vi "the end - 복사본.vi"() -> ()   [LabVIEW 2011]
uses:
  <vilib>/NXT/Block Support/NXT_InputPort.ctl
  <vilib>/NXT/Subs/MotorOutput.ctl
  <vilib>/NXT/Dual Mode Library/Waits/Wait_Num.vi
  <vilib>/NXT/Dual Mode Library/Motors/MotorOn.vi
panel:
  out "Yes / No":bool
  in  "터치 센서 (port 2)":T1 caption="Port (Port 1)" items=["Port 1", "Port 2", "Port 3", "Port 4"]
  in  "소나 센서 (port 3)":T1=3 caption="Port (Port 4)" items=["Port 1", "Port 2", "Port 3", "Port 4"]
  in  "회전 각도 4":i32=180
  in  "회전 각도 3":i32=180
  in  "회전 포트 4":T2=3 items=["Port A"=0, "Port B"=1, "Port C"=2, "Ports A & B"=4, "Ports A & C"=5, "Ports B & C"=6, "All Ports"=3]
  in  "회전 포트 3":T2=3 items=["Port A"=0, "Port B"=1, "Port C"=2, "Ports A & B"=4, "Ports A & C"=5, "Ports B & C"=6, "All Ports"=3]
  in  "후진 시간 2":sgl=1.0
  in  "빛 센서 (port 1)":T1=2 caption="Port (Port 3)" items=["Port 1", "Port 2", "Port 3", "Port 4"]
  in  "정지":bool
  in  "회전 각도 2":i32=180
  in  "회전 각도 1":i32=180
  in  "회전 포트 1":T2=3 items=["Port A"=0, "Port B"=1, "Port C"=2, "Ports A & B"=4, "Ports A & C"=5, "Ports B & C"=6, "All Ports"=3]
  in  "회전 포트 2":T2=3 items=["Port A"=0, "Port B"=1, "Port C"=2, "Ports A & B"=4, "Ports A & C"=5, "Ports B & C"=6, "All Ports"=3]
  in  "후진 시간":sgl=1.0
  in  "Power (100)":i32=75
  in  "Output Port (All Ports)":T2=3 items=["Port A"=0, "Port B"=1, "Port C"=2, "Ports A & B"=4, "Ports A & C"=5, "Ports B & C"=6, "All Ports"=3]
  in  "빛 센서 (port 4)":T1=2 caption="Port (Port 3)" items=["Port 1", "Port 2", "Port 3", "Port 4"]
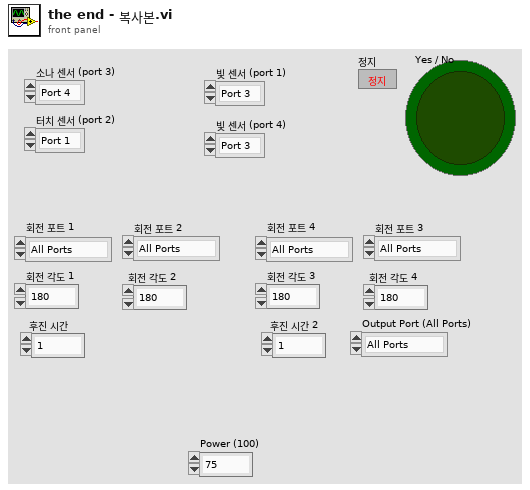
[diagram p1: front panel]
types:
  T1 = typedef "NXT_InputPort.ctl" = u8
  T2 = typedef "MotorOutput.ctl" = u8
  T3 = typedef "LVHSConnector.ctl" = cluster{"Hardware":string, "Flattened String":string}
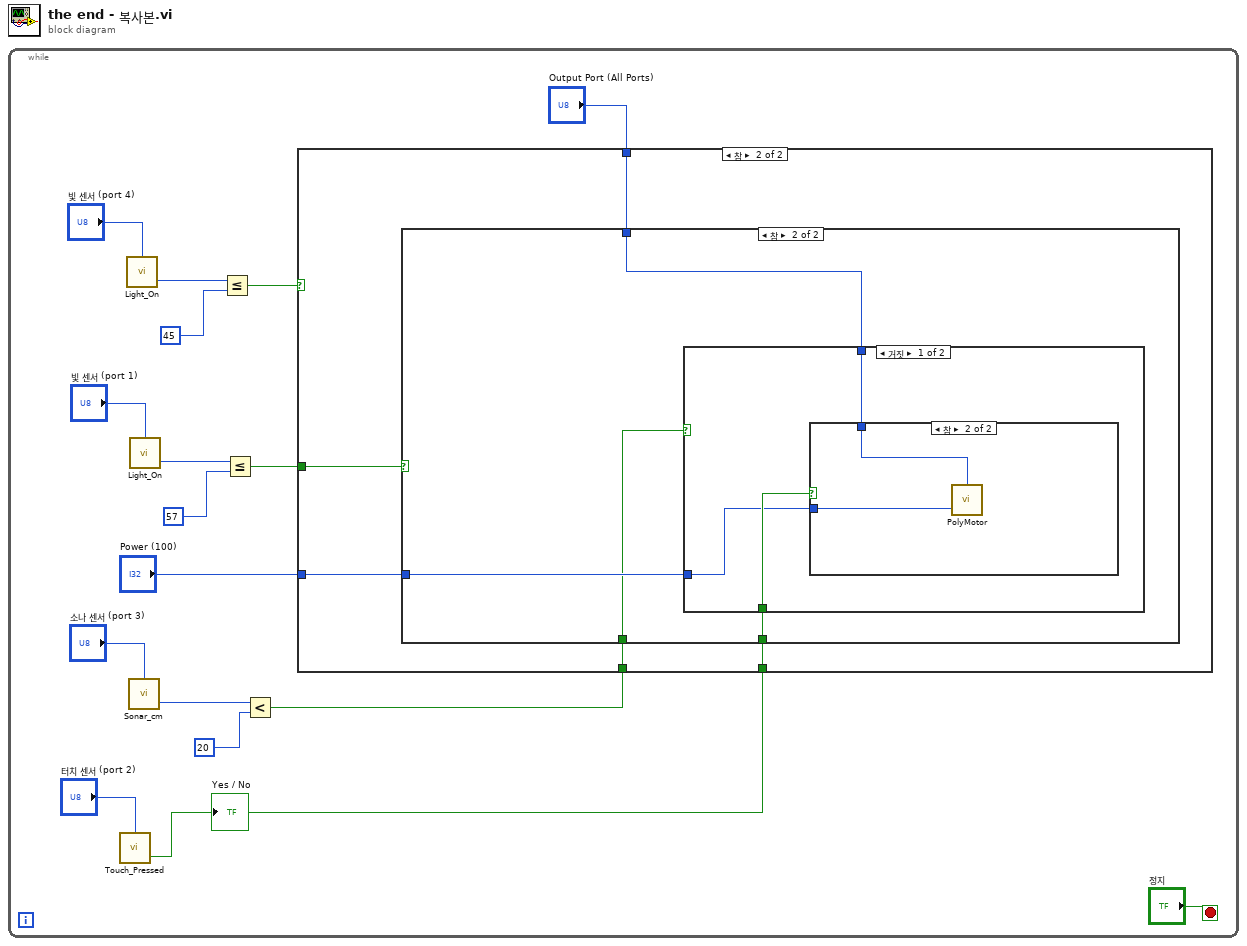
[diagram p0: block diagram]
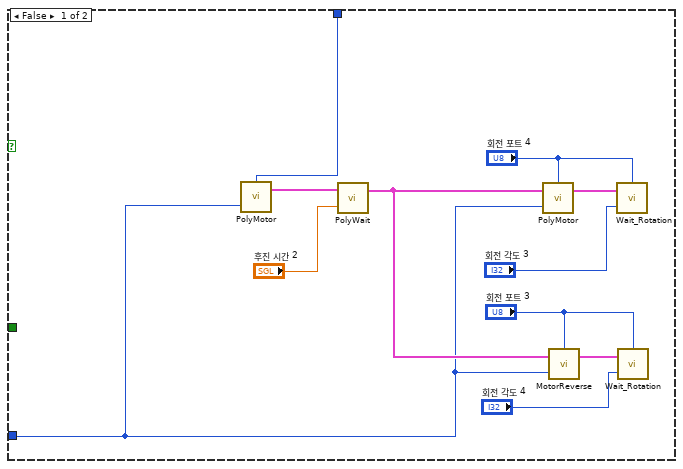
[diagram p2: hidden frame]
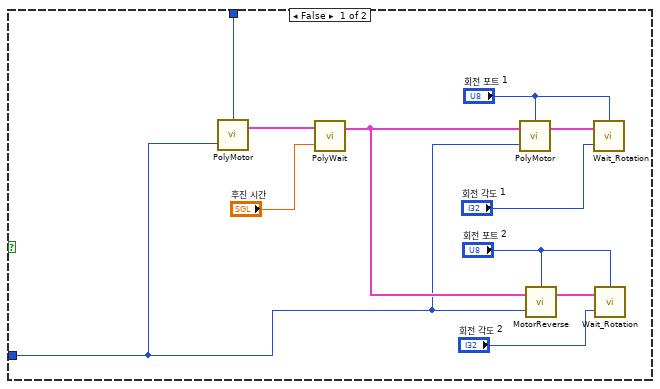
[diagram p3: hidden frame]
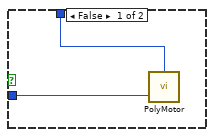
[diagram p4: hidden frame]
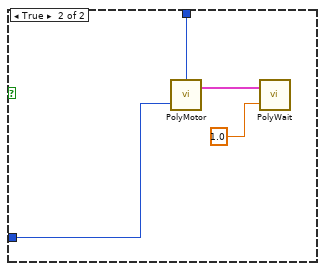
[diagram p5: hidden frame]
diagram:
  n1 = while {
    stop <- "정지" stop-if-true
    n2 = call <vilib>:"Touch_Pressed.vi"("Port (Port 1)"="터치 센서 (port 2)") -> ("Yes / No"=w1:bool)  [unwired: 2 in, 1 out]
    "Yes / No" <- w1
    n3 = call <vilib>:"Light_On.vi"("Port (Port 3)"="빛 센서 (port 4)") -> ("Scaled Value"=w15:i16)  [unwired: 2 in, 1 out]
    n4 = call <vilib>:"Sonar_cm.vi"("Port (Port 4)"="소나 센서 (port 3)") -> ("Distance (cm)"=w7:i16)  [unwired: 2 in, 1 out]
    n5 = call <vilib>:"Light_On.vi"("Port (Port 3)"="빛 센서 (port 1)") -> ("Scaled Value"=w11:i16)  [unwired: 2 in, 1 out]
    n6 = Less Or Equal?(x=w15, y=i16 45) -> (x <= y?=w14:bool)
    n7 = Less Or Equal?(x=w11, y=i16 57) -> (x <= y?=w9:bool)
    n8 = Less?(x=w7, y=i16 20) -> (x < y?=w6:bool)
    n9 = case shown="참" w14 {
      tunnel: w9 -> [_ w33]
      tunnel: "Output Port (All Ports)" -> [w19 w32]
      tunnel: "Power (100)" -> [w18 w31]
      tunnel: w6 -> [_ w30]
      tunnel: w1 -> [_ w29]
      frame False {
        n10 = call-poly <vilib>:"PolyMotor.vi"("Power (75)"=w18, "Output Port (All Ports)"=w19) -> ("NXT"=w20:T3)  [unwired: 2 in]
        n11 = call-poly <vilib>:"PolyWait.vi"("Time (1 sec)"="후진 시간 2", "NXT"=w20) -> ("NXT"=w22:T3)  [unwired: 2 in]
        n12 = call-poly <vilib>:"PolyMotor.vi"("Power (75)"=w18, "NXT"=w22, "Output Port (All Ports)"="회전 포트 4") -> ("NXT"=w21:T3)  [unwired: 1 in]
        n13 = call <vilib>:"MotorReverse.vi"("Power (75)"=w18, "NXT"=w22, "Output Port (All Ports)"="회전 포트 3") -> ("NXT"=w23:T3)  [unwired: 1 in]
        n14 = call <vilib>:"Wait_Rotation.vi"("Position Change (180)"="회전 각도 3", "NXT"=w21, "Port (Port A)"="회전 포트 4") -> ()  [unwired: 1 in, 1 out]
        n15 = call <vilib>:"Wait_Rotation.vi"("Position Change (180)"="회전 각도 4", "NXT"=w23, "Port (Port A)"="회전 포트 3") -> ()  [unwired: 1 in, 1 out]
      }
      frame True {
        n16 = case shown="참" w33 {
          tunnel: w32 -> [w35 w48]
          tunnel: w31 -> [w34 w47]
          tunnel: w30 -> [_ w46]
          tunnel: w29 -> [_ w45]
          frame False {
            n17 = call-poly <vilib>:"PolyMotor.vi"("Power (75)"=w34, "Output Port (All Ports)"=w35) -> ("NXT"=w36:T3)  [unwired: 2 in]
            n18 = call-poly <vilib>:"PolyWait.vi"("Time (1 sec)"="후진 시간", "NXT"=w36) -> ("NXT"=w38:T3)  [unwired: 2 in]
            n19 = call-poly <vilib>:"PolyMotor.vi"("Power (75)"=w34, "NXT"=w38, "Output Port (All Ports)"="회전 포트 1") -> ("NXT"=w37:T3)  [unwired: 1 in]
            n20 = call <vilib>:"MotorReverse.vi"("Power (75)"=w34, "NXT"=w38, "Output Port (All Ports)"="회전 포트 2") -> ("NXT"=w39:T3)  [unwired: 1 in]
            n21 = call <vilib>:"Wait_Rotation.vi"("Position Change (180)"="회전 각도 1", "NXT"=w37, "Port (Port A)"="회전 포트 1") -> ()  [unwired: 1 in, 1 out]
            n22 = call <vilib>:"Wait_Rotation.vi"("Position Change (180)"="회전 각도 2", "NXT"=w39, "Port (Port A)"="회전 포트 2") -> ()  [unwired: 1 in, 1 out]
          }
          frame True {
            n23 = case shown="거짓" w46 {
              tunnel: w48 -> [w50 w59]
              tunnel: w47 -> [w49 w56]
              tunnel: w45 -> [w51 _]
              frame False {
                n24 = case shown="참" w51 {
                  tunnel: w50 -> [w53 w55]
                  tunnel: w49 -> [w52 w54]
                  frame False {
                    n25 = call-poly <vilib>:"PolyMotor.vi"("Power (75)"=w52, "Output Port (All Ports)"=w53) -> ()  [unwired: 2 in, 1 out]
                  }
                  frame True {
                    n26 = call-poly <vilib>:"PolyMotor.vi"("Power (75)"=w54, "Output Port (All Ports)"=w55) -> ()  [unwired: 2 in, 1 out]
                  }
                }
              }
              frame True {
                n27 = call-poly <vilib>:"PolyMotor.vi"("Power (75)"=w56, "Output Port (All Ports)"=w59) -> ("NXT"=w58:T3)  [unwired: 2 in]
                n28 = call-poly <vilib>:"PolyWait.vi"("Time (1 sec)"=sgl 1.0, "NXT"=w58) -> ()  [unwired: 2 in, 1 out]
              }
            }
          }
        }
      }
    }
  }
